vi "Event Handler.vi"(8 "error in (no error)":errorcluster, 10 "Stop Event Handler":refnum<user-event>, 11 "MCLBSelection in":refnum<class "MulticolumnListboxSelection.lvclass">) -> (0 "error out":errorcluster)   [LabVIEW 2015, in "MulticolumnListboxSelection.lvclass"]
doc: "The <b>Event Handler VI</b> is a dynamic dispatch VI that should be overwritten if events are needed to create the enhanced QControl. \n\nBy inheriting from the main Control.lvclass the overwritten <b>Event Handler VI</b> will be launched asynchronously in the initialization of the QControl.\n<b> </b> <b> </b>\n©2016 Q Software Innovations, LLC (QSI)\nwritten by Quentin Alldredge\nproduced in LabVIEW 2015\n\nsupport@qsoftwareinnovations.com\nwww.qsoftwareinnovations.com\n\nAll rights reserved.\n\nRedistribution and use in source and binary forms, with or without modification, are permitted provided that the following conditions are met:\n\n * Redistributions of source code must retain the above copyright notice, this list of conditions and the following disclaimer.\n * Redistributions in binary form must reproduce the above copyright notice, this list of conditions and the following disclaimer in the documentation and/or other materials provided with the distribution.\n * Neither the name of Q Software Innovations, LLC. nor the names of its contributors may be used to endorse or promote products derived from this software without specific prior written permission.\n\nTHIS SOFTWARE IS PROVIDED BY THE COPYRIGHT HOLDERS AND CONTRIBUTORS \"AS IS\" AND ANY EXPRESS OR IMPLIED WARRANTIES, INCLUDING, BUT NOT LIMITED TO, THE IMPLIED WARRANTIES OF MERCHANTABILITY AND FITNESS FOR A PARTICULAR PURPOSE ARE DISCLAIMED. IN NO EVENT SHALL THE COPYRIGHT OWNER OR CONTRIBUTORS BE LIABLE FOR ANY DIRECT, INDIRECT, INCIDENTAL, SPECIAL, EXEMPLARY, OR CONSEQUENTIAL DAMAGES (INCLUDING, BUT NOT LIMITED TO, PROCUREMENT OF SUBSTITUTE GOODS OR SERVICES; LOSS OF USE, DATA, OR PROFITS; OR BUSINESS INTERRUPTION) HOWEVER CAUSED AND ON ANY THEORY OF LIABILITY, WHETHER IN CONTRACT, STRICT LIABILITY, OR TORT (INCLUDING NEGLIGENCE OR OTHERWISE) ARISING IN ANY WAY OUT OF THE USE OF THIS SOFTWARE, EVEN IF ADVISED OF THE POSSIBILITY OF SUCH DAMAGE."
uses:
  MulticolumnListboxSelection.lvclass
  MulticolumnListboxSelection.lvclass/MulticolumnListboxSelection.ctl
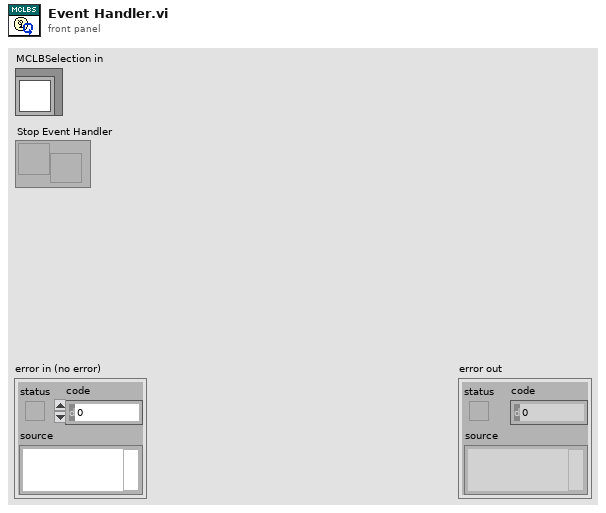
[diagram p1: front panel]
types:
  T1 = typedef "LVPoint32TypeDef.ctl" = cluster{"Horizontal":i32, "Vertical":i32}
  T2 = typedef "LVRowAndColumnTypeDef.ctl" = cluster{"Row":i32, "Column":i32}
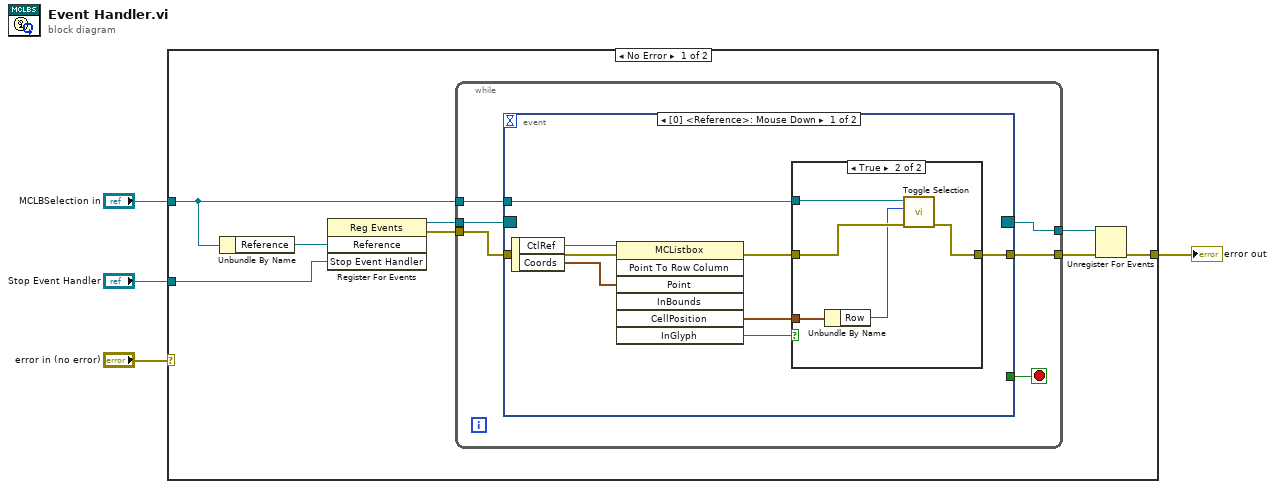
[diagram p0: block diagram]
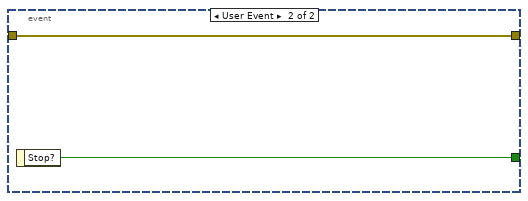
[diagram p3: hidden frame]
diagram:
  n1 = case shown="No Error" "error in (no error)" {
    selector: "error in (no error)" -> [_ w35]
    tunnel: [w7 w35] -> w3
    tunnel: "MCLBSelection in" -> [w8 _]
    tunnel: "Stop Event Handler" -> [w5 _]
    frame No Error {
      n2 = Unbundle By Name(w8) -> ("Reference"=w6:refnum<vi>)
      n3 = register-events(w6, w5) -> (reference out=w9:refnum<event-registration>, error out=w10:errorcluster)  [unwired: 2 in]
      n4 = while {
        tunnel: w9 -> [w18]
        tunnel: w10 -> [w16]
        tunnel: [w15] -> w11
        tunnel: [w13] -> w12
        tunnel: w8 -> [w17]
        stop <- w14 stop-if-true
        n5 = event shown="[0] <Reference>: Mouse Down" {
          selector: w18 -> [_ _]
          dyn-events: [_ _] -> w13
          timeout: _ -> [_ _]
          tunnel: w17 -> [w24 _]
          tunnel: w16 -> [w22 w34]
          tunnel: [w20 w34] -> w15
          tunnel: [_ w33] -> w14
          event Mouse Down {
            n6 = event-data() -> ("CtlRef"=w26:refnum<vi>, "Coords"=w25:T1)  [unwired: 1 in]
            n7 = invoke class="MCListbox" method="Point To Row Column"(reference=w26, error in=w22, "Point"=w25) -> (error out=w21:errorcluster, "CellPosition"=w23:T2, "InGlyph"=w19:bool)  [unwired: 4 in, 4 out]
            n8 = case shown="True" w19 {
              tunnel: w24 -> [_ w31]
              tunnel: w23 -> [_ w32]
              tunnel: w21 -> [w27 w30]
              tunnel: [w27 w29] -> w20
              frame False {
              }
              frame True {
                n9 = Unbundle By Name(w32) -> ("Row"=w28:i32)
                n10 = call-dynamic "Toggle Selection.vi"("error in (no error)"=w30, "Item Index"=w28, "MCLBSelection in"=w31) -> ("error out"=w29:errorcluster)  [unwired: 7 in, 1 out]
              }
            }
          }
          event User Event {
            n11 = event-data() -> ("Stop?"=w33:bool)  [unwired: 1 in]
          }
        }
      }
      n12 = Unregister For Events(event registration refnum=w12, error in=w11) -> (error out=w7:errorcluster)
    }
    frame Error {
    }
  }
  "error out" <- w3
